vi "Set_file_path.vi"(8 "error in (no error)":errorcluster caption="错误输入（无错误）") -> (0 "error out":errorcluster caption="错误输出", 3 "appended path":path)   [LabVIEW 2018]
uses:
  Global.vi
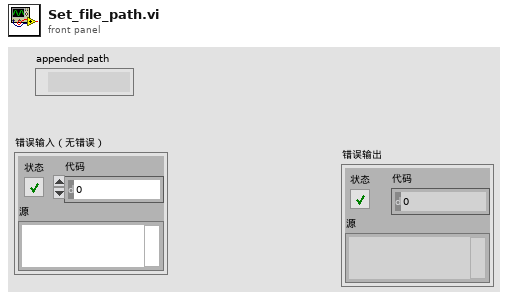
[diagram p1: front panel]
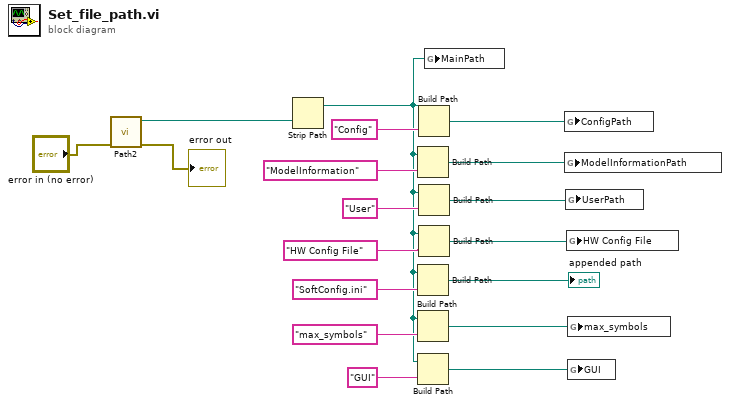
[diagram p0: block diagram]
diagram:
  n1 = call "Path2.vi"("error in (no error)"="error in (no error)") -> ("error out"=→"error out":errorcluster, "拆分的路径"=w10:path)  [unwired: 9 in]
  n2 = Strip Path(path=w10) -> (stripped path=w3:path)  [unwired: 1 out]
  n3 = Build Path(base path=w3, name or relative path="ModelInformation") -> (appended path=w12:path)
  n4 = Build Path(base path=w3, name or relative path="SoftConfig.ini" ("名称或相对路径")) -> (appended path=→"appended path":path)
  n5 = Build Path(base path=w3, name or relative path="max_symbols" ("名称或相对路径")) -> (appended path=w7:path)
  n6 = Build Path(base path=w3, name or relative path="GUI" ("名称或相对路径")) -> (appended path=w4:path)
  n7 = Build Path(base path=w3, name or relative path="Config" ("名称或相对路径")) -> (appended path=w13:path)
  n8 = Build Path(base path=w3, name or relative path="User") -> (appended path=w14:path)
  n9 = Build Path(base path=w3, name or relative path="HW Config File") -> (appended path=w15:path)
  n10 = global write "Global.vi" "MainPath"(w3) -> ()
  n11 = global write "Global.vi" "ConfigPath"(w13) -> ()
  n12 = global write "Global.vi" "ModelInformationPath"(w12) -> ()
  n13 = global write "Global.vi" "UserPath"(w14) -> ()
  n14 = global write "Global.vi" "HW Config File"(w15) -> ()
  n15 = global write "Global.vi" "max_symbols"(w7) -> ()
  n16 = global write "Global.vi" "GUI"(w4) -> ()
